vi "read_attributes.vi"(8 "error in (no error)":errorcluster, 11 "RadiusNeighborsClassifier in":refnum<class "RadiusNeighborsClassifier.lvclass">) -> (0 "error out":errorcluster, 2 "attributes":T1, 3 "RadiusNeighborsClassifier out":refnum<class "RadiusNeighborsClassifier.lvclass">)   [LabVIEW 2020, in "RadiusNeighborsClassifier.lvclass"]
uses:
  RadiusNeighborsClassifier.lvclass
  Controls/radius_neighbors_classifier_attributes.ctl
  RadiusNeighborsClassifier.lvclass/RadiusNeighborsClassifier.ctl
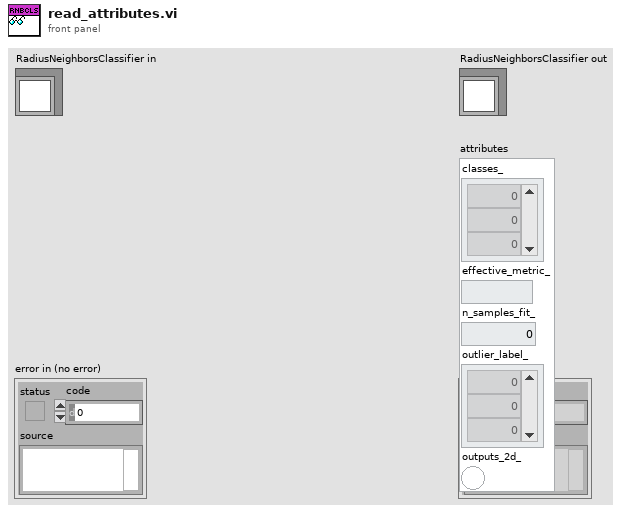
[diagram p1: front panel]
types:
  T1 = typedef "radius_neighbors_classifier_attributes.ctl" = cluster{"classes_":dbl[], "effective_metric_":string, "n_samples_fit_":dbl, "outlier_label_":dbl[], "outputs_2d_":bool}
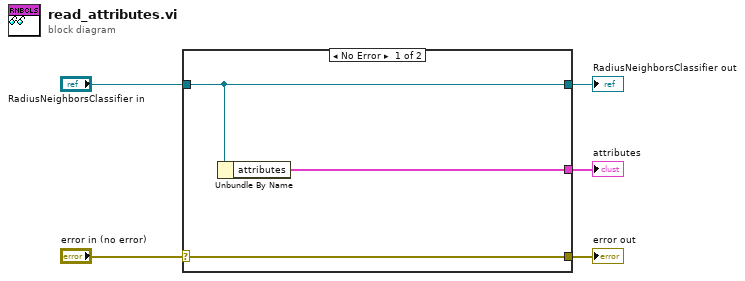
[diagram p0: block diagram]
diagram:
  n1 = case shown="No Error" "error in (no error)" {
    selector: "error in (no error)" -> [w8 w9]
    tunnel: [w8 w9] -> w4
    tunnel: [w7 w10] -> w2
    tunnel: "RadiusNeighborsClassifier in" -> [w7 w10]
    tunnel: [w6 _] -> w1
    frame No Error {
      n2 = Unbundle By Name(w7) -> ("attributes"=w6:T1)
    }
    frame Error {
    }
  }
  "error out" <- w4
  "RadiusNeighborsClassifier out" <- w2
  "attributes" <- w1
